vi "SetDistFromWallAuto.vi"() -> ()   [LabVIEW 2020]
panel:
  in  "Timeout":dbl
  in  "Distance":dbl
  in  "MaxSpeed":dbl
  out "Done":bool
  in  "error in":errorcluster
  out "error out":errorcluster
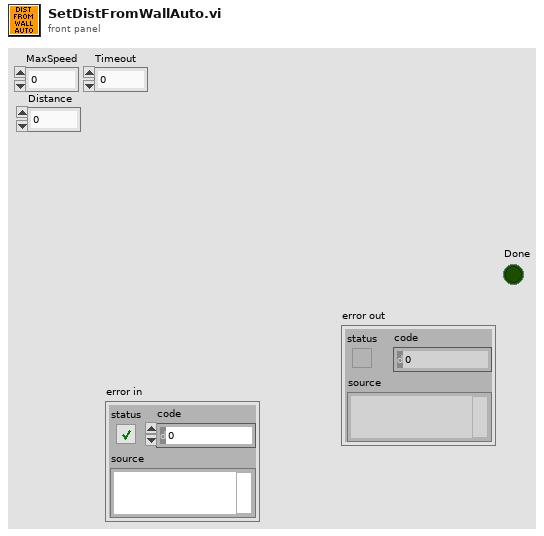
[diagram p1: front panel]
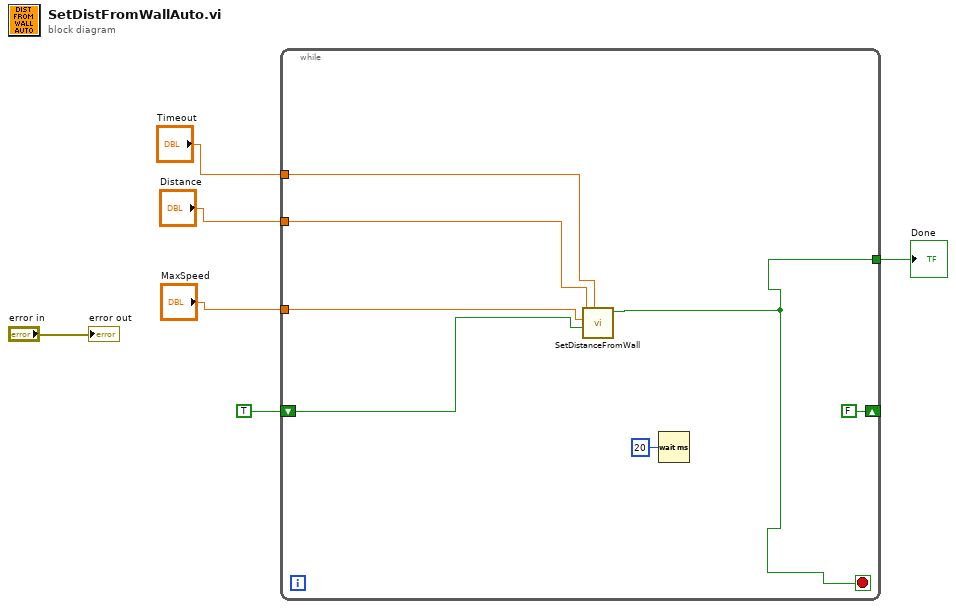
[diagram p0: block diagram]
diagram:
  n1 = while {
    tunnel: [w11] -> w5
    tunnel: "MaxSpeed" -> [w9]
    tunnel: "Distance" -> [w8]
    tunnel: "Timeout" -> [w7]
    shift-right: [FALSE] -> _
    shift-left: TRUE -> [w10]
    stop <- w11 stop-if-true
    n2 = call "SetDistanceFromWall.vi"("Timeout"=w7, "Initation?"=w10, "MaxSpeed"=w9, "Distance"=w8) -> ("Finished"=w11:bool)  [unwired: 5 in, 2 out]
    n3 = Wait (ms)(milliseconds to wait=u32 20) -> ()  [unwired: 1 out]
  }
  "Done" <- w5
  "error out" <- "error in"
